vi "firealert_labview.vi"() -> ()   [LabVIEW 2018]
panel:
  out "SMOKE":u8(slide) scale=0.0..1.0
  out "FIRE INDICATOR":bool
  in  "VISA resource name":refnum<visa-resource-name>
  out "HUMIDITY":dbl(graph)
  out "SMOKE":dbl(graph)
  out "TEPMPERATURE":dbl(graph)
  in  "Table Control":string[][](table)=[["DATA", "TIME", "TEMP", "SMOKE", "HUM", "ID"]]
  out "HUMIDITY":dbl(knob) scale=0.0..100.0
  out "HUMIDITY":bool
  out "SMOKE":bool
  out "TEMPERATURE":bool
  out "TEMPERATURE":dbl(slide) scale=0.0..100.0
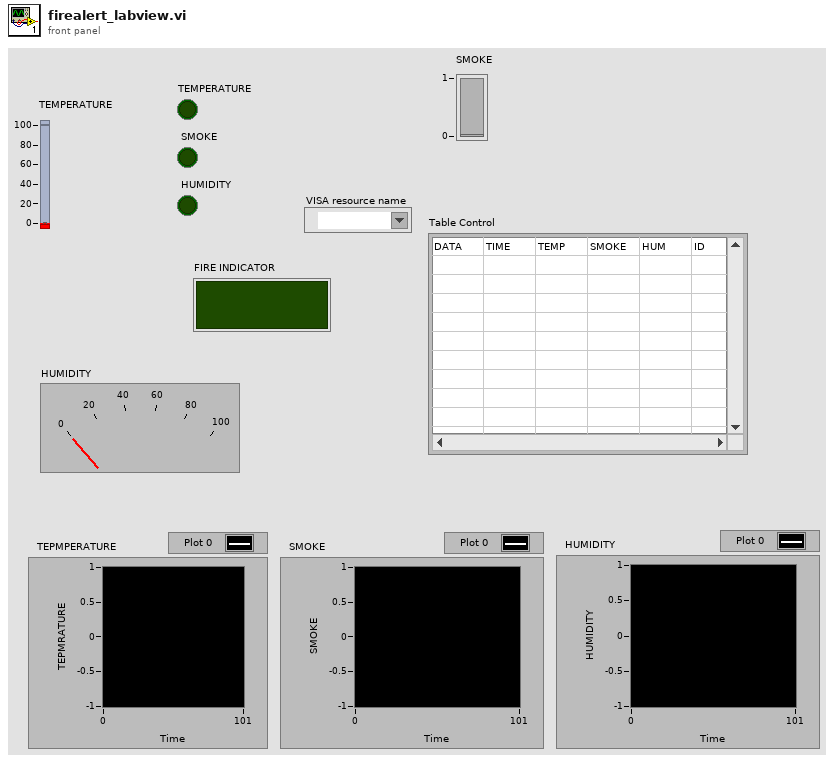
[diagram p1: front panel]
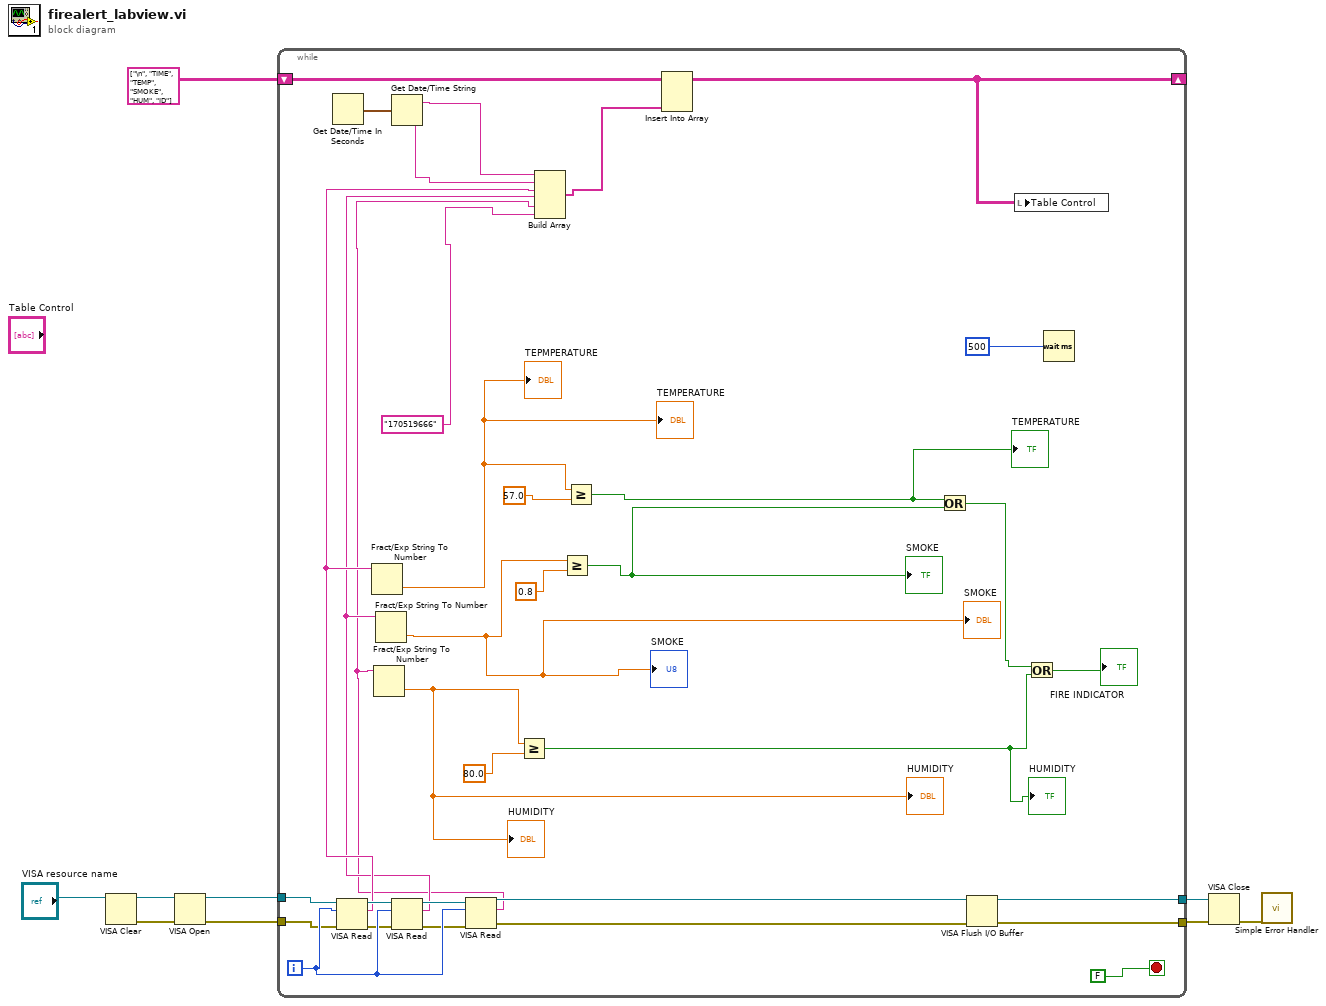
[diagram p0: block diagram]
diagram:
  n1 = VISA Clear(VISA resource name="VISA resource name") -> (VISA resource name out=w8:refnum<visa-resource-name>, error out=w6:errorcluster)  [unwired: 1 in]
  n2 = VISA Open(error in (no error)=w6, VISA resource name=w8) -> (VISA resource name=w7:refnum<visa-resource-name>, error out=w5:errorcluster)  [unwired: 3 in]
  n3 = while {
    tunnel: w7 -> [w40]
    tunnel: w5 -> [w37]
    tunnel: [w32] -> w4
    tunnel: [w31] -> w3
    shift-right: [w17] -> _
    shift-left: string[][] [["\n", "TIME", "TEMP", "SMOKE", "HUM", "ID"]] ("Table Control") -> [w18]
    i -> [w41]
    stop <- FALSE stop-if-true
    n4 = Get Date/Time In Seconds() -> (seconds since 1Jan1904=w43:timestamp)
    n5 = VISA Read(VISA resource name=w40, byte count=w41, error in (no error)=w37) -> (VISA resource name out=w39:refnum<visa-resource-name>, read buffer=w14:string, error out=w36:errorcluster)  [unwired: 1 out]
    n6 = Fract/Exp String To Number(string=w14) -> (number=w24:dbl)  [unwired: 3 in, 1 out]
    "TEMPERATURE" <- w24
    "TEPMPERATURE" <- w24
    n7 = Get Date/Time String(seconds (now)=w43) -> (date string=w16:string, time string=w15:string)  [unwired: 2 in]
    n8 = VISA Read(VISA resource name=w39, byte count=w41, error in (no error)=w36) -> (VISA resource name out=w38:refnum<visa-resource-name>, read buffer=w13:string, error out=w35:errorcluster)  [unwired: 1 out]
    n9 = Fract/Exp String To Number(string=w13) -> (number=w28:dbl)  [unwired: 3 in, 1 out]
    "SMOKE" <- w28
    "SMOKE" <- w28
    n10 = VISA Read(VISA resource name=w38, byte count=w41, error in (no error)=w35) -> (VISA resource name out=w34:refnum<visa-resource-name>, read buffer=w12:string, error out=w33:errorcluster)  [unwired: 1 out]
    n11 = Fract/Exp String To Number(string=w12) -> (number=w21:dbl)  [unwired: 3 in, 1 out]
    "HUMIDITY" <- w21
    "HUMIDITY" <- w21
    n12 = Greater Or Equal?(x=w21, y=80.0) -> (x >= y?=w20:bool)
    "HUMIDITY" <- w20
    n13 = Build Array(w16, w15, w14, w13, w12, "170519666") -> (w10:string[])
    n14 = Greater Or Equal?(x=w28, y=0.8) -> (x >= y?=w27:bool)
    "SMOKE" <- w27
    n15 = Greater Or Equal?(x=w24, y=57.0) -> (x >= y?=w25:bool)
    "TEMPERATURE" <- w25
    n16 = Insert Into Array "Insert Into Array"(array=w18, new element=w10) -> (w17:string[][])  [unwired: 2 in]
    n17 = Or(x=w25, y=w27) -> (x .or. y?=w26:bool)
    n18 = VISA Flush I/O Buffer(VISA resource name=w34, error in (no error)=w33) -> (VISA resource name out=w32:refnum<visa-resource-name>, error out=w31:errorcluster)  [unwired: 1 in]
    n19 = local write "Table Control"(w17) -> ()
    n20 = Or(x=w26, y=w20) -> (x .or. y?=→"FIRE INDICATOR":bool)
    n21 = Wait (ms)(milliseconds to wait=500) -> ()  [unwired: 1 out]
  }
  n22 = VISA Close(VISA resource name=w4, error in (no error)=w3) -> (error out=w1:errorcluster)
  n23 = call <vilib>:"Simple Error Handler.vi"("error in (no error)"=w1) -> ()  [unwired: 4 in, 5 out]
